vi "MPM_Get_Logging_Status.vi"(8 "error in (no error)":errorcluster, 11 ".NET Reference in":refnum<k24>) -> (0 "error out":errorcluster, 1 "count out":i32, 2 "status out":i32, 3 "Reference out":refnum<k24>)   [LabVIEW 2017]
uses:
  D:/test/ILSTS/LV_IL_Sample/DLL/InstrumentDLL.dll
  DLL/InstrumentDLL.dll
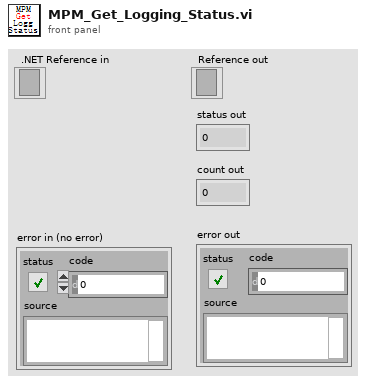
[diagram p1: front panel]
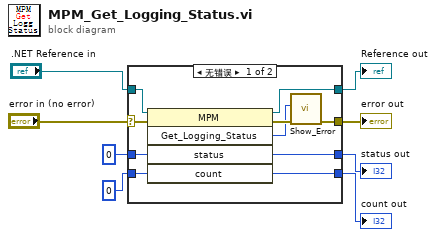
[diagram p0: block diagram]
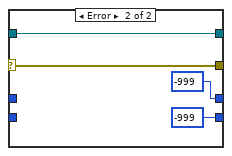
[diagram p2: hidden frame]
diagram:
  n1 = case shown="无错误" "error in (no error)" {
    selector: "error in (no error)" -> [w9 w22]
    tunnel: [w18 -999 ("count")] -> w8
    tunnel: [w17 -999 ("status")] -> w7
    tunnel: ".NET Reference in" -> [w16 w19]
    tunnel: [w15 w19] -> w5
    tunnel: 0 ("status") -> [w14 _]
    tunnel: 0 ("count") -> [w13 _]
    tunnel: [w10 w22] -> w2
    frame No Error {
      n2 = invoke class="MPM" method="Get_Logging_Status"(reference=w16, error in=w9, "status"=w14, "count"=w13) -> (reference out=w15:refnum<k24>, error out=w12:errorcluster, "Get_Logging_Status"=w11:i32, "status"=w17:i32, "count"=w18:i32)  [unwired: 1 in]
      n3 = call "Show_Error.vi"("error in (no error)"=w12, "Error"=w11) -> ("error out"=w10:errorcluster)  [unwired: 9 in]
    }
    frame Error {
    }
  }
  "count out" <- w8
  "status out" <- w7
  "Reference out" <- w5
  "error out" <- w2
